vi "Execute ShowLabelsOfClusterElements.vi"(6 "Mouse Position":T1, 8 "User VI Ref":refnum<vi>, 9 "Menu Item Tag Suffix":string, 10 "Remaining Items":refnum<vi>[](array[refnum]), 11 "Affected Items":T2) -> (0 "Fail transaction?":bool)   [LabVIEW 2017]
doc: "This VI is part of a plug-in for modifying the LabVIEW shortcut menus. This is the execute VI which is called when the shortcut menu is chosen by the user. It performs the action of the selected menu item."
uses:
  <resource>/plugins/PopupMenus/edit time panel and diagram/Expand Cluster Constant.llb/Expand Cluster Constant.ctl
  <vilib>/Utility/miscctls.llb/LVPositionTypeDef.ctl
panel:
  # "All controls on this panel except \"Affected Items\" have been locked to prevent accidental edits. Changing the control names or types, other than the elements of the \"Affected Items\" cluster will make the VI unusable as a menu plugin.\n\nSee Context Help for each control for details about its use."
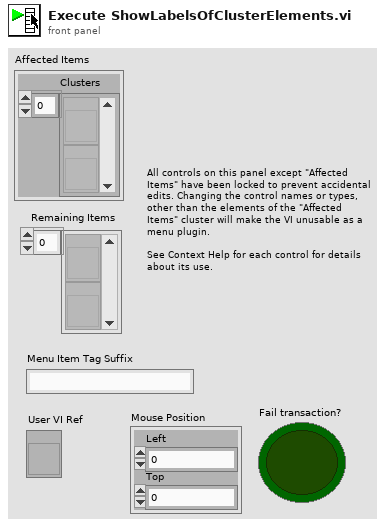
[diagram p1: front panel]
types:
  T1 = typedef "LVPositionTypeDef.ctl" = cluster{"Left":i32, "Top":i32}
  T2 = typedef "Expand Cluster Constant.ctl" = cluster{"Clusters":refnum<vi>[]}
  T3 = enum32{"None", "Size to Fit", "Arrange Horizontally", "Arrange Vertically"}
  T4 = typedef "LVRectTypeDef.ctl" = cluster{"Left":i16, "Top":i16, "Right":i16, "Bottom":i16}
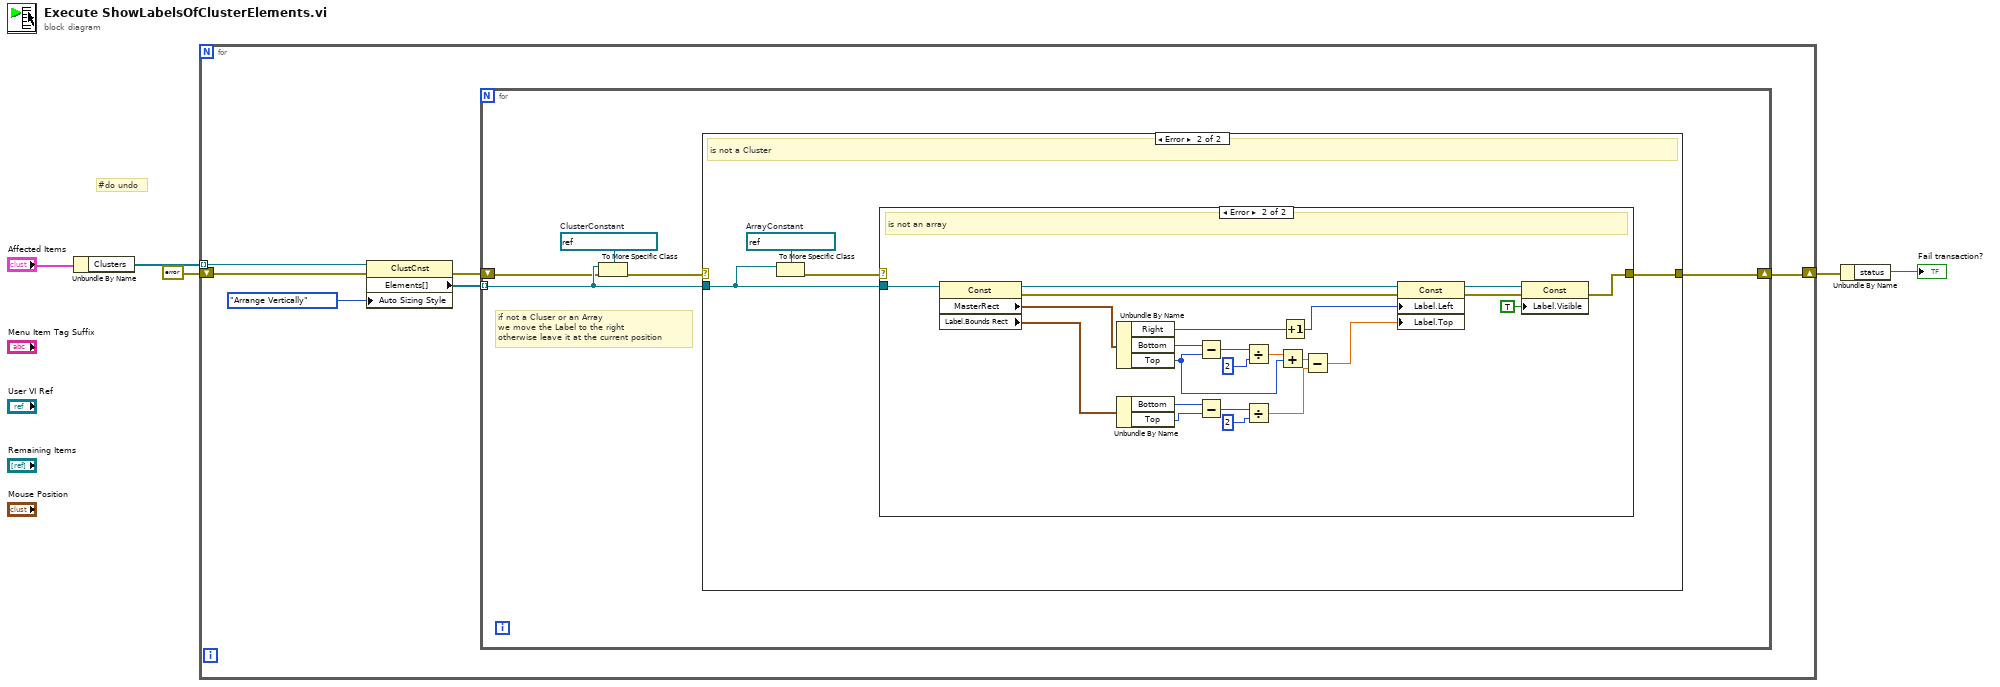
[diagram p0: block diagram]
diagram:
  # "#do undo"
  n1 = Unbundle By Name("Affected Items") -> ("Clusters"=w4:refnum<vi>[])
  n2 = for {
    tunnel: w4 -> [w11] mode=indexing
    shift-right: [w6] -> w2
    shift-left: errorcluster {"status"=FALSE, "code"=0, "source"=""} ("error out") -> [w8]
    n3 = property class="ClustCnst"(reference=w11, error in=w8, "Auto Sizing Style"=T3."Arrange Vertically") -> (error out=w9:errorcluster, "Elements[]"=w10:refnum<vi>[])  [unwired: 1 out]
    n4 = for {
      tunnel: w10 -> [w14] mode=indexing
      shift-right: [w16] -> w6
      shift-left: w9 -> [w13]
      w15 = refnum<vi> refnum  # ClusterConstant
      # "if not a Cluser or an Array\nwe move the Label to the right\notherwise leave it at the current position"
      n5 = To More Specific Class(target class=w15, reference=w14, error in=w13) -> (error out=w12:errorcluster)  [unwired: 1 out]
      n6 = case shown="Error" w12 {
        selector: w12 -> [w17 _]
        tunnel: [w17 w21] -> w16
        tunnel: w14 -> [_ w19]
        frame No Error {
        }
        frame Error {
          w20 = refnum<vi> refnum  # ArrayConstant
          # "is not a Cluster"
          n7 = To More Specific Class(target class=w20, reference=w19) -> (error out=w18:errorcluster)  [unwired: 1 in, 1 out]
          n8 = case shown="Error" w18 {
            selector: w18 -> [w22 _]
            tunnel: [w22 w23] -> w21
            tunnel: w19 -> [_ w26]
            frame No Error {
            }
            frame Error {
              # "is not an array"
              n9 = property class="Const"(reference=w26) -> (reference out=w33:refnum<vi>, error out=w28:errorcluster, "MasterRect"=w44:T4, "Label.Bounds Rect"=w36:T4)  [unwired: 1 in]
              n10 = Unbundle By Name(w44) -> ("Right"=w43:i16, "Bottom"=w38:i16, "Top"=w37:i16)
              n11 = Unbundle By Name(w36) -> ("Bottom"=w35:i16, "Top"=w34:i16)
              n12 = Subtract(x=w38, y=w37) -> (x-y=w42:i16)
              n13 = Subtract(x=w35, y=w34) -> (x-y=w31:i16)
              n14 = Divide(x=w42, y=i16 2) -> (x/y=w40:dbl)
              n15 = Divide(x=w31, y=i16 2) -> (x/y=w30:dbl)
              n16 = Add(x=w40, y=w37) -> (x+y=w39:dbl)
              n17 = Increment(x=w43) -> (x+1=w29:i16)
              n18 = Subtract(x=w39, y=w30) -> (x-y=w27:dbl)
              n19 = property class="Const"(reference=w33, error in=w28, "Label.Left"=w29, "Label.Top"=w27) -> (reference out=w25:refnum<vi>, error out=w24:errorcluster)
              n20 = property class="Const"(reference=w25, error in=w24, "Label.Visible"=TRUE) -> (error out=w23:errorcluster)  [unwired: 1 out]
            }
          }
        }
      }
    }
  }
  n21 = Unbundle By Name(w2) -> ("status"=→"Fail transaction?":bool)
